vi "Search and Replace String.vi"(8 "error in (no error)":errorcluster, 9 "Replace Str":string="ABCSN", 10 "FindStr":string="flash_once.bat SN", 11 "originalTex":string="@echo off\nsetlocal enabledelayedexpansion\n\nREM ========= 用户可配置区 =========\nset RFP_DIR=C:\\Program Files (x86)\\Renesas Electronics\\Programming Tools\\Renesas Flash Programmer V3.16\nset RFP_EXE=%RFP_DIR%\\RFPV3.exe\nset RFP_CONSOLE=%RFP_DIR%\\RFPV3.Console.exe\n\nset PROJECT=D:\\Alvin\\1.Project\\5.ZhiRuiJia\\Flash\\RFP_Auto\\Project\\k7001.rpj\nREM 固件已配置在 .rpj 内，这里默认不再单独指定 /file\nset FIRMWARE=\nset LOG_DIR=D:\\Alvin\\1.Project\\5.ZhiRuiJia\\Flash\\RFP_Auto\\Logs\nset RETRY=2\nREM 可选：如果你只有一台E2 Lite，通常不需要指定tool序列号\nset TOOL_SN=\nREM 示例：set TOOL_SN=xxxxxxxxx\nREM =================================\n\nif not exist \"%LOG_DIR%\" mkdir \"%LOG_DIR%\"\n\nREM SN 可由扫码枪/上位机传入：flash_once.bat SNABCSN\nset SN=%1\nif \"%SN%\"==\"\" set SN=NO_SN\n\nREM 时间戳（yyyyMMdd_HHmmss）\nfor /f %%i in ('powershell -NoProfile -Command \"Get-Date -Format yyyyMMdd_HHmmss\"') do set TS=%%i\n\nset LOG_FILE=%LOG_DIR%\\%SN%_%TS%.log\n\necho [INFO] SN=%SN%\necho [INFO] Project=%PROJECT%\nif not \"%FIRMWARE%\"==\"\" echo [INFO] Firmware=%FIRMWARE%\necho [INFO] Log=%LOG_FILE%\necho.\n\nREM 参数拼接\nset COMMON_ARGS=/silent \"%PROJECT%\" /command epv /log \"%LOG_FILE%\"\nif not \"%FIRMWARE%\"==\"\" set COMMON_ARGS=%COMMON_ARGS% /file \"%FIRMWARE%\"\nif not \"%TOOL_SN%\"==\"\" set COMMON_ARGS=%COMMON_ARGS% /tool %TOOL_SN%\n\nset /a COUNT=0\n\n:RETRY_LOOP\nset /a COUNT+=1\necho [INFO] Attempt !COUNT! ...\n\nREM 优先用 RFPV3.exe /silent\n\"%RFP_EXE%\" %COMMON_ARGS%\nset RC=%ERRORLEVEL%\n\necho [INFO] ExitCode=%RC%\n\nif \"%RC%\"==\"0\" goto PASS\n\nif !COUNT! LEQ %RETRY% (\n    echo [WARN] Programming failed, retrying...\n    timeout /t 2 >nul\n    goto RETRY_LOOP\n)\n\ngoto FAIL\n\n:PASS\nfor /f %%i in ('powershell -NoProfile -Command \"Get-Date -Format yyyyMMdd_HHmmss\"') do set END_TS=%%i\necho [INFO] EndTime=%END_TS%\necho [PASS] %SN% %TS% >> \"%LOG_DIR%\\summary_pass.txt\"\necho SUCCESS\nexit /b 0\n\n:FAIL\nfor /f %%i in ('powershell -NoProfile -Command \"Get-Date -Format yyyyMMdd_HHmmss\"') do set END_TS=%%i\necho [INFO] EndTime=%END_TS%\necho [FAIL] %SN% %TS% ExitCode=%RC% >> \"%LOG_DIR%\\summary_fail.txt\"\necho FAIL\nexit /b 1\n") -> (0 "error out":errorcluster, 3 "output Str":string="@echo off\nsetlocal enabledelayedexpansion\n\nREM ========= 用户可配置区 =========\nset RFP_DIR=C:\\Program Files (x86)\\Renesas Electronics\\Programming Tools\\Renesas Flash Programmer V3.16\nset RFP_EXE=%RFP_DIR%\\RFPV3.exe\nset RFP_CONSOLE=%RFP_DIR%\\RFPV3.Console.exe\n\nset PROJECT=D:\\Alvin\\1.Project\\5.ZhiRuiJia\\Flash\\RFP_Auto\\Project\\k7001.rpj\nREM 固件已配置在 .rpj 内，这里默认不再单独指定 /file\nset FIRMWARE=\nset LOG_DIR=D:\\Alvin\\1.Project\\5.ZhiRuiJia\\Flash\\RFP_Auto\\Logs\nset RETRY=2\nREM 可选：如果你只有一台E2 Lite，通常不需要指定tool序列号\nset TOOL_SN=\nREM 示例：set TOOL_SN=xxxxxxxxx\nREM =================================\n\nif not exist \"%LOG_DIR%\" mkdir \"%LOG_DIR%\"\n\nREM SN 可由扫码枪/上位机传入：flash_once.bat SNABCSN\nset SN=%1\nif \"%SN%\"==\"\" set SN=NO_SN\n\nREM 时间戳（yyyyMMdd_HHmmss）\nfor /f %%i in ('powershell -NoProfile -Command \"Get-Date -Format yyyyMMdd_HHmmss\"') do set TS=%%i\n\nset LOG_FILE=%LOG_DIR%\\%SN%_%TS%.log\n\necho [INFO] SN=%SN%\necho [INFO] Project=%PROJECT%\nif not \"%FIRMWARE%\"==\"\" echo [INFO] Firmware=%FIRMWARE%\necho [INFO] Log=%LOG_FILE%\necho.\n\nREM 参数拼接\nset COMMON_ARGS=/silent \"%PROJECT%\" /command epv /log \"%LOG_FILE%\"\nif not \"%FIRMWARE%\"==\"\" set COMMON_ARGS=%COMMON_ARGS% /file \"%FIRMWARE%\"\nif not \"%TOOL_SN%\"==\"\" set COMMON_ARGS=%COMMON_ARGS% /tool %TOOL_SN%\n\nset /a COUNT=0\n\n:RETRY_LOOP\nset /a COUNT+=1\necho [INFO] Attempt !COUNT! ...\n\nREM 优先用 RFPV3.exe /silent\n\"%RFP_EXE%\" %COMMON_ARGS%\nset RC=%ERRORLEVEL%\n\necho [INFO] ExitCode=%RC%\n\nif \"%RC%\"==\"0\" goto PASS\n\nif !COUNT! LEQ %RETRY% (\n    echo [WARN] Programming failed, retrying...\n    timeout /t 2 >nul\n    goto RETRY_LOOP\n)\n\ngoto FAIL\n\n:PASS\nfor /f %%i in ('powershell -NoProfile -Command \"Get-Date -Format yyyyMMdd_HHmmss\"') do set END_TS=%%i\necho [INFO] EndTime=%END_TS%\necho [PASS] %SN% %TS% >> \"%LOG_DIR%\\summary_pass.txt\"\necho SUCCESS\nexit /b 0\n\n:FAIL\nfor /f %%i in ('powershell -NoProfile -Command \"Get-Date -Format yyyyMMdd_HHmmss\"') do set END_TS=%%i\necho [INFO] EndTime=%END_TS%\necho [FAIL] %SN% %TS% ExitCode=%RC% >> \"%LOG_DIR%\\summary_fail.txt\"\necho FAIL\nexit /b 1\r\n")   [LabVIEW 2024]
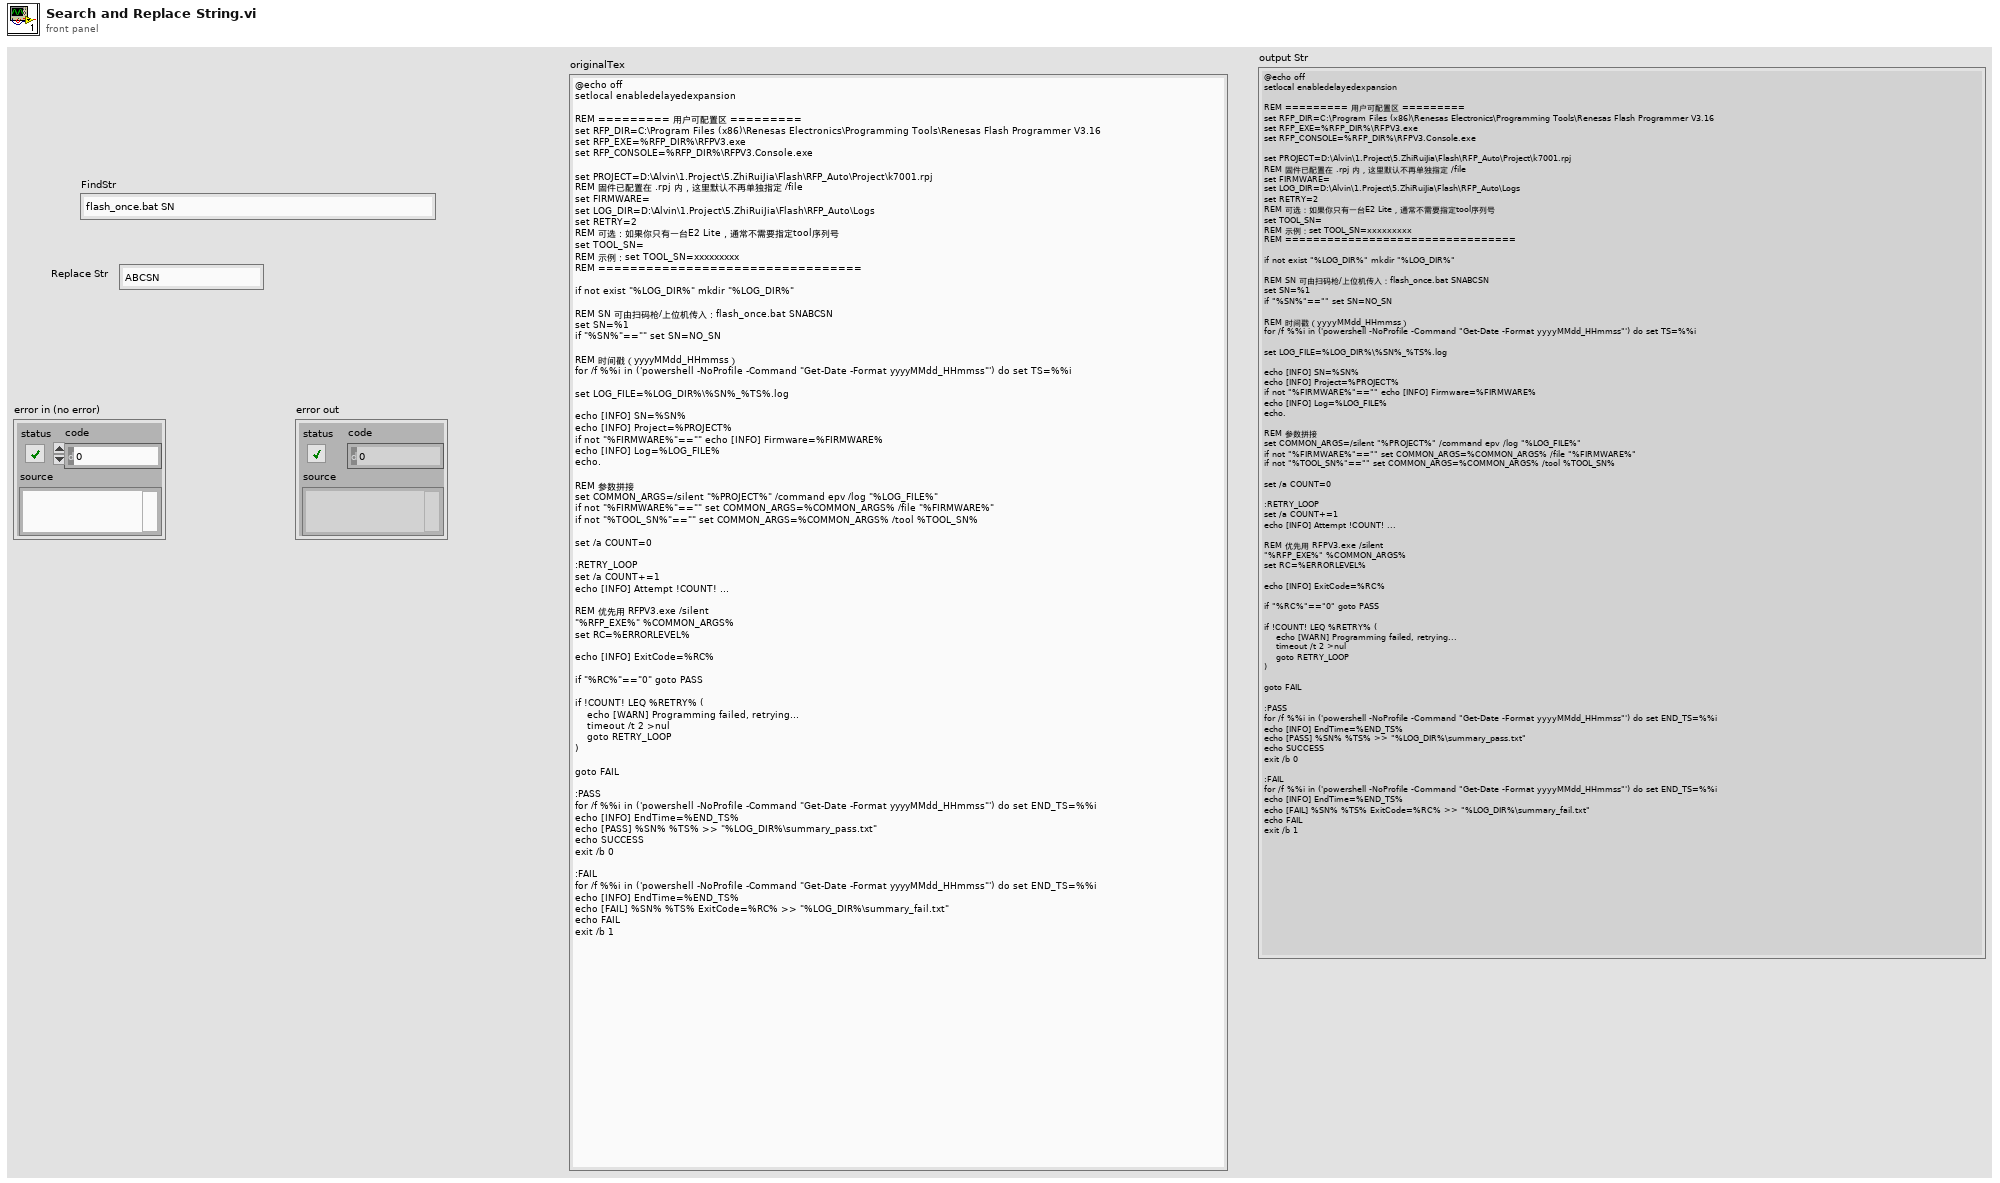
[diagram p1: front panel]
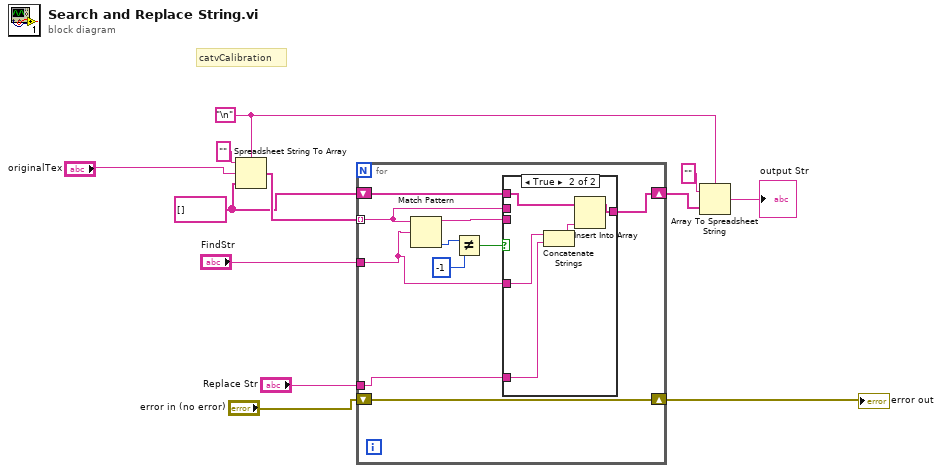
[diagram p0: block diagram]
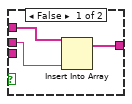
[diagram p2: hidden frame]
diagram:
  w9 = string[] []
  w5 = "\n"
  # "catvCalibration"
  n1 = Spreadsheet String To Array(delimiter (Tab)=w5, format string="", spreadsheet string="originalTex", array type (2D Dbl)=w9) -> (array=w11:string[])
  n2 = for {
    tunnel: w11 -> [w16] mode=indexing
    tunnel: "FindStr" -> [w15]
    shift-right: [w19] -> w7
    shift-left: w9 -> [w20]
    tunnel: "Replace Str" -> [w18]
    shift-right: [w17] -> w2
    shift-left: "error in (no error)" -> [w17]
    n3 = Match Pattern(string=w16, regular expression=w15) -> (before substring=w14:string, offset past match=w13:i32)  [unwired: 1 in, 2 out]
    n4 = Not Equal?(x=w13, y=-1) -> (x != y?=w21:bool)
    n5 = case shown="True" w21 {
      tunnel: w16 -> [w24 _]
      tunnel: w20 -> [w25 w29]
      tunnel: [w23 w27] -> w19
      tunnel: w18 -> [_ w30]
      tunnel: w15 -> [_ w26]
      tunnel: w14 -> [_ _]
      frame False {
        n6 = Insert Into Array(array=w25, new element=w24) -> (w23:string[])  [unwired: 1 in]
      }
      frame True {
        n7 = Concatenate Strings(w26, w30) -> (w28:string)
        n8 = Insert Into Array(array=w29, new element=w28) -> (w27:string[])  [unwired: 1 in]
      }
    }
  }
  "error out" <- w2
  n9 = Array To Spreadsheet String(delimiter (Tab)=w5, array=w7, 3:"" ("format string")) -> (spreadsheet string=→"output Str":string)
